vi "decoupling_test.vi"() -> ()   [LabVIEW 2013]
panel:
  out "Max err re-decoupled":sgl format="%#_3g"
  out "max err I/O":sgl format="%#_3g"
  out "Re-decoupled":sgl[](array[numeric]) format="%#_3g"
  out "Decoupled":sgl[](array[numeric]) format="%#_3g"
  out "Output":sgl[](array[numeric]) format="%#_3g"
  in  "Input":sgl[](array[numeric])
  # "----------XY----------"
  # "----------RxRy----------"
  # "Z"
  # "Rz"
  # "----------XY----------"
  # "----------RxRy----------"
  # "Z"
  # "Rz"
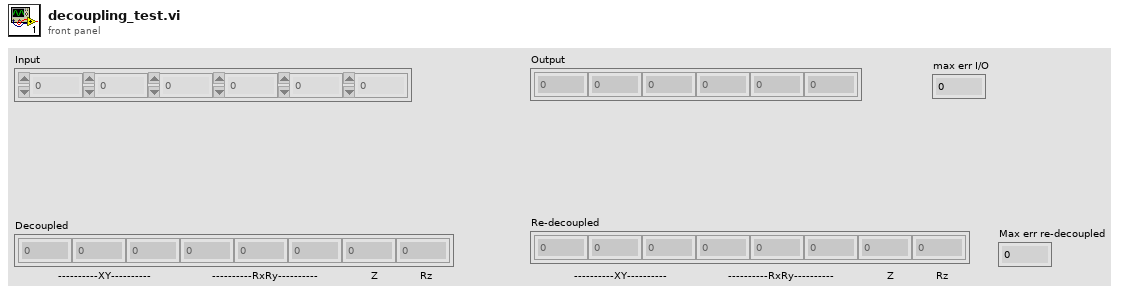
[diagram p1: front panel]
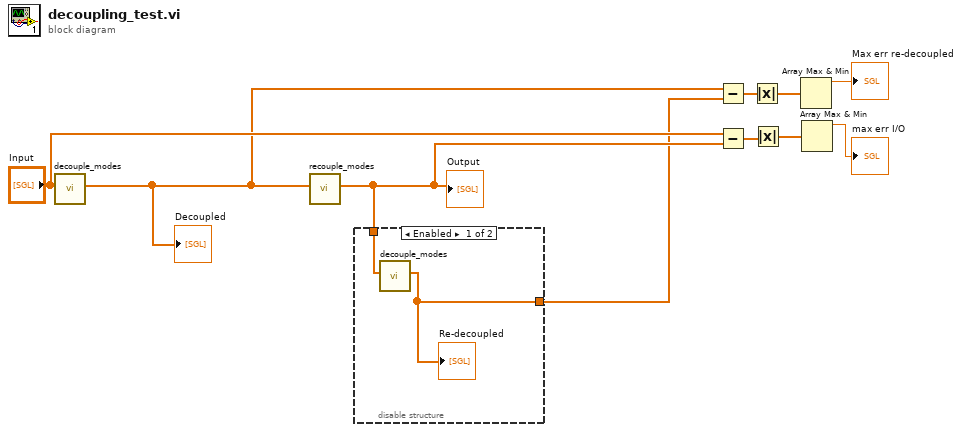
[diagram p0: block diagram]
diagram:
  n1 = call "decouple_modes.vi"("Input"="Input") -> ("Decoupled"=w8:sgl[])  [unwired: 10 in]
  "Decoupled" <- w8
  n2 = call "recouple_modes.vi"("Decoupled"=w8) -> ("Output"=w9:sgl[])  [unwired: 10 in]
  "Output" <- w9
  n3 = disable-structure shown="Enabled" {
    disable-tunnel: w9 -> [w12 _]
    disable-tunnel: [w11 _] -> w7
    frame Enabled {
      n4 = call "decouple_modes.vi"("Input"=w12) -> ("Decoupled"=w11:sgl[])  [unwired: 10 in]
      "Re-decoupled" <- w11
    }
    frame Disabled {
    }
  }
  n5 = Subtract(x=w8, y=w7) -> (x-y=w6:sgl[])
  n6 = Subtract(x="Input", y=w9) -> (x-y=w4:sgl[])
  n7 = Absolute Value(x=w6) -> (abs(x)=w5:sgl[])
  n8 = Absolute Value(x=w4) -> (abs(x)=w3:sgl[])
  n9 = Array Max & Min(array=w5) -> (max value=→"Max err re-decoupled":sgl)  [unwired: 3 out]
  n10 = Array Max & Min(array=w3) -> (max value=→"max err I/O":sgl)  [unwired: 3 out]
